vi "TahomaTestModern2023.vi"() -> ()   [LabVIEW 2023]
panel:
  in  "Boolean":bool
  in  "Tab Control":enum32{"Tahoma 15 pt", "TEST"}(tab)
  in  "Tahoma 15 pt":string="abcdefghijklmnopqrstuvwxyzßüöä\nABCDEFGHIJKLMNOPQRSTUVWXYZÜÖÄ\n1234567890\n1111111111\n^´+#<,.-°!\"§$%&/()=?`*'>;:_²³{[]}\\~|\n\nThe quick brown fox jumps over the lazy dog\n\nLorem ipsum dolor sit amet, consectetur adipiscing elit, sed do eiusmod tempor incididunt ut labore et dolore magna aliqua. Ut enim ad minim veniam, quis nostrud exercitation ullamco laboris nisi ut aliquip ex ea commodo consequat. Duis aute irure dolor in reprehenderit in voluptate velit esse cillum dolore eu fugiat nulla pariatur. Excepteur sint occaecat cupidatat non proident, sunt in culpa qui officia deserunt mollit anim id est laborum."
  in  "Arial 15 pt":string="abcdefghijklmnopqrstuvwxyzßüöä\nABCDEFGHIJKLMNOPQRSTUVWXYZÜÖÄ\n1234567890\n1111111111\n^´+#<,.-°!\"§$%&/()=?`*'>;:_²³{[]}\\~|\n\nThe quick brown fox jumps over the lazy dog\n\nLorem ipsum dolor sit amet, consectetur adipiscing elit, sed do eiusmod tempor incididunt ut labore et dolore magna aliqua. Ut enim ad minim veniam, quis nostrud exercitation ullamco laboris nisi ut aliquip ex ea commodo consequat. Duis aute irure dolor in reprehenderit in voluptate velit esse cillum dolore eu fugiat nulla pariatur. Excepteur sint occaecat cupidatat non proident, sunt in culpa qui officia deserunt mollit anim id est laborum."
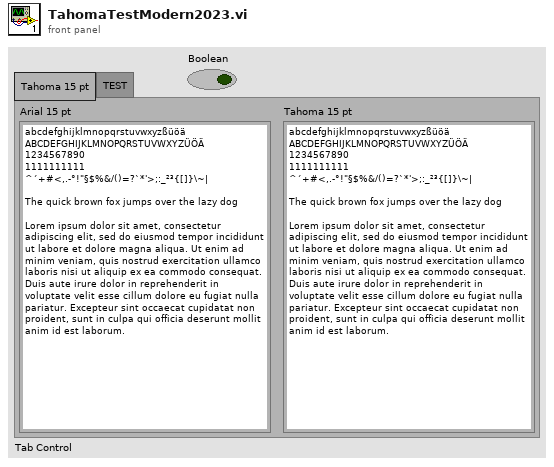
[diagram p1: front panel]
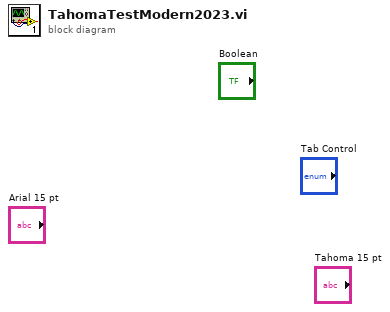
[diagram p0: block diagram]
diagram:
